vi "set_origin.vi"(8 "error in (no error)":errorcluster, 11 "DL090202ScanHead in":refnum<class "ScanHeadDL090202.lvclass">) -> (0 "error out":errorcluster, 3 "DL090202ScanHead out":refnum<class "ScanHeadDL090202.lvclass">)   [LabVIEW 2010, in "ScanHeadDL090202.lvclass"]
uses:
  ScanHeadDL090202.lvclass
  ScanHeadDL090202.lvclass/ScanHeadDL090202.ctl
  common/classes/ErrorController/ErrorController/class_data.vi
  common/classes/SpaceVector/SpaceVector/SpaceVector.lvclass
  Stage/GenericStage/GenericStage/GenericStage.lvclass
  Stage/GenericStage/GenericStage/trigger_enum.ctl
  common/classes/ErrorController/ErrorController/ErrorController.lvclass
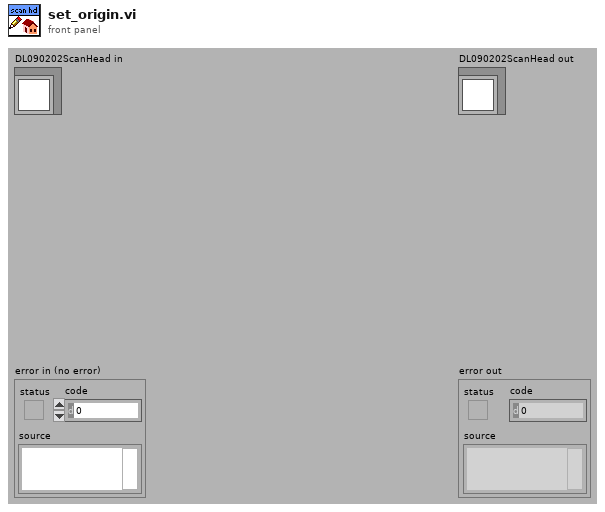
[diagram p1: front panel]
types:
  T1 = typedef "GenericStage.lvclass/trigger_enum.ctl" = enum16{"NULL", "initialise", "terminate", "move", "update position", "set origin", "return to origin"}
  T2 = typedef "ScanHeadDL090202.lvclass/translation_mode_enum.ctl" = enum16{"scan signal offset", "stage"}
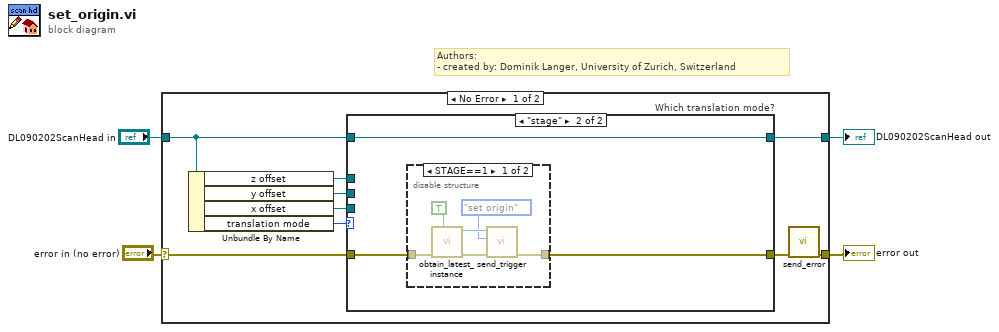
[diagram p0: block diagram]
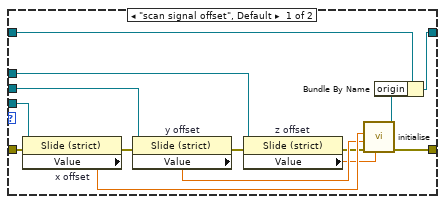
[diagram p2: hidden frame]
diagram:
  # "Authors: \n- created by: Dominik Langer, University of Zurich, Switzerland"
  n1 = case shown="No Error" "error in (no error)" {
    selector: "error in (no error)" -> [w5 w39]
    tunnel: [w7 w39] -> w2
    tunnel: [w9 w38] -> w1
    tunnel: "DL090202ScanHead in" -> [w11 w38]
    frame No Error {
      n2 = Unbundle By Name(w11) -> ("z offset"=w10:refnum<vi>, "y offset"=w12:refnum<vi>, "x offset"=w13:refnum<vi>, "translation mode"=w6:T2)
      n3 = case "Which translation mode?" shown="\"stage\"" w6 {
        tunnel: w13 -> [w26 _]
        tunnel: w12 -> [w24 _]
        tunnel: w11 -> [w23 w28]
        tunnel: w10 -> [w20 _]
        tunnel: [w16 w28] -> w9
        tunnel: [w15 w29] -> w8
        tunnel: w5 -> [w14 w30]
        frame "scan signal offset", Default {
          n4 = property on="x offset" class="Slide (strict)"(reference=w26, error in=w14) -> (error out=w25:errorcluster, "Value"=w22:dbl[unit])  [unwired: 1 out]
          n5 = property on="y offset" class="Slide (strict)"(reference=w24, error in=w25) -> (error out=w19:errorcluster, "Value"=w21:dbl[unit])  [unwired: 1 out]
          n6 = property on="z offset" class="Slide (strict)"(reference=w20, error in=w19) -> (error out=w18:errorcluster, "Value"=w17:dbl[unit])  [unwired: 1 out]
          n7 = call "initialise.vi"("z"=w17, "error in (no error)"=w18, "y"=w21, "x"=w22) -> ("error out"=w15:errorcluster, "SpaceVector out"=w27:refnum<class "SpaceVector.lvclass">)  [unwired: 6 out]
          n8 = Bundle By Name(cluster=w23, "origin"=w27) -> (w16:refnum<class "ScanHeadDL090202.lvclass">)
        }
        frame "stage" {
          n9 = disable-structure shown="STAGE==1" {
            disable-tunnel: w30 -> [w32 w37]
            disable-tunnel: [w31 w37] -> w29
            frame condition #0 {
              n10 = call "obtain_latest_instance.vi"("quick, but maybe outdated?"=TRUE, "error in (no error)"=w32) -> ("error out"=w36:errorcluster, "GenericStage out"=w34:refnum<class "GenericStage.lvclass">)  [unwired: 8 in]
              n11 = call-dynamic "send_trigger.vi"("error in (no error)"=w36, "trigger"=trigger_enum."set origin", "GenericStage in"=w34) -> ("error out"=w31:errorcluster)  [unwired: 7 in, 1 out]
            }
            frame condition #1 (active) {
            }
          }
        }
      }
      n12 = call "send_error.vi"("error in (no error)"=w8) -> ("error out"=w7:errorcluster)  [unwired: 10 in]
    }
    frame Error {
    }
  }
  "error out" <- w2
  "DL090202ScanHead out" <- w1
